vi "GE 5565PIORC.DMA.Wait for Done.vi"(7 "wait mode (polling)":T1, 8 "error in (no error)":errorcluster, 10 "timeout ms (1000)":u32=1000, 11 "GE 5565PIORC in":refnum<class "GE 5565PIORC.lvclass">) -> (0 "error out":errorcluster, 2 "timed out?":bool, 3 "GE 5565PIORC out":refnum<class "GE 5565PIORC.lvclass">)   [LabVIEW 2020, in "GE 5565PIORC.lvclass"]
doc: "Waits the specified <b>timeout</b> period for the GE 5565PIORC to assert an interrupt for a completed DMA transfer."
uses:
  GE 5565PIORC.lvclass
  Typedefs/GE 5565PIORC.Typedef.DMA Wait Mode.ctl
  GE 5565PIORC.lvclass/GE 5565PIORC.ctl
  Properties/Registers/GE 5565PIORC.Registers.Local Configuration.Read.vi
  Properties/Registers/GE 5565PIORC.Registers.Local Configuration.Read (U8).vi
  Properties/Registers/GE 5565PIORC.Registers.Local Configuration.Write.vi
  Properties/Registers/GE 5565PIORC.Registers.Local Configuration.Write (U8).vi
  GE 5565PIORC.Bit Manipulation.Set Bit.vi
  GE 5565PIORC.Bit Manipulation.Set Bit (U8).vi
  GE 5565PIORC.DMA.Is Done.vi
  <vilib>/Utility/error.llb/Clear Errors.vi
  GE 5565PIORC.Registers.Read.vi
  GE 5565PIORC.Registers.Read (U8).vi
  GE 5565PIORC.Registers.Write.vi
  GE 5565PIORC.Registers.Write (U8).vi
  Properties/Registers/GE 5565PIORC.Registers.DMACSR0.Channel 0 Inactive.Get.vi
  GE 5565PIORC.Bit Manipulation.Get Bit.vi
  GE 5565PIORC.Bit Manipulation.Get Bit (U8).vi
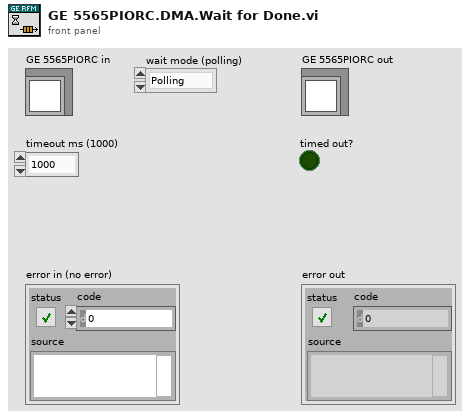
[diagram p1: front panel]
types:
  T1 = typedef "GE 5565PIORC.lvclass/GE 5565PIORC.Typedef.DMA Wait Mode.ctl" = enum16{"Polling", "Interrupt"}
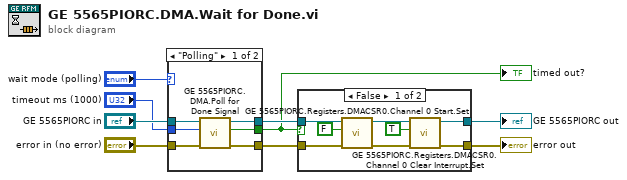
[diagram p0: block diagram]
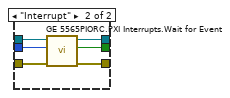
[diagram p2: hidden frame]
diagram:
  n1 = case shown="\"Polling\"" "wait mode (polling)" {
    tunnel: "error in (no error)" -> [w13 w21]
    tunnel: "GE 5565PIORC in" -> [w15 w20]
    tunnel: "timeout ms (1000)" -> [w12 w19]
    tunnel: [w10 w18] -> w6
    tunnel: [w14 w17] -> w5
    tunnel: [w11 w16] -> w2
    frame "Polling" {
      n2 = call "GE 5565PIORC.DMA.Poll for Done Signal.vi"("error in (no error)"=w13, "timeout ms (1000)"=w12, "GE 5565PIORC in"=w15) -> ("error out"=w10:errorcluster, "timed out?"=w11:bool, "GE 5565PIORC out"=w14:refnum<class "GE 5565PIORC.lvclass">)  [unwired: 6 in]
    }
    frame "Interrupt" {
      n3 = call "GE 5565PIORC.PXI Interrupts.Wait for Event.vi"("error in (no error)"=w21, "timeout ms (1000)"=w19, "GE 5565PIORC in"=w20) -> ("error out"=w18:errorcluster, "timed out?"=w16:bool, "GE 5565PIORC out"=w17:refnum<class "GE 5565PIORC.lvclass">)  [unwired: 6 in]
    }
  }
  "timed out?" <- w2
  n4 = case shown="False" w2 {
    tunnel: w6 -> [w29 w30]
    tunnel: w5 -> [w28 w31]
    tunnel: [w23 w31] -> w4
    tunnel: [w22 w30] -> w3
    frame False {
      n5 = call "GE 5565PIORC.Registers.DMACSR0.Channel 0 Start.Set.vi"("error in (no error)"=w29, "Channel 0 Start"=FALSE, "GE 5565PIORC in"=w28) -> ("error out"=w25:errorcluster, "GE 5565PIORC out"=w26:refnum<class "GE 5565PIORC.lvclass">)  [unwired: 7 in]
      n6 = call "GE 5565PIORC.Registers.DMACSR0.Channel 0 Clear Interrupt.Set.vi"("error in (no error)"=w25, "Channel 0 Clear Interrupt"=TRUE, "GE 5565PIORC in"=w26) -> ("error out"=w22:errorcluster, "GE 5565PIORC out"=w23:refnum<class "GE 5565PIORC.lvclass">)  [unwired: 7 in]
    }
    frame True {
    }
  }
  "GE 5565PIORC out" <- w4
  "error out" <- w3
